vi "Clear Buffers.vi"(8 "error in (no error)":errorcluster, 11 "TDCManager":T1) -> (0 "error out":errorcluster, 3 "TDCManager":T1)   [LabVIEW 2016, in "HPTDC Driver Library.lvlib"]
uses:
  HPTDC Driver Library.lvlib
  Typedefs/TDCManager.ctl
  C:/Users/CRT Controller/CRTC Labview Application/Source/HPTDC Driver Library Folder/Library files/hptdc_net4_3.7.0_x64.dll
  hptdc_net4_3.7.0_x64.dll
panel:
  out "Succes?":bool
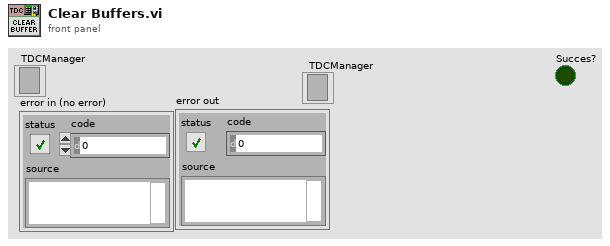
[diagram p1: front panel]
types:
  T1 = typedef "HPTDC Driver Library.lvlib/TDCManager.ctl" = refnum<k24>
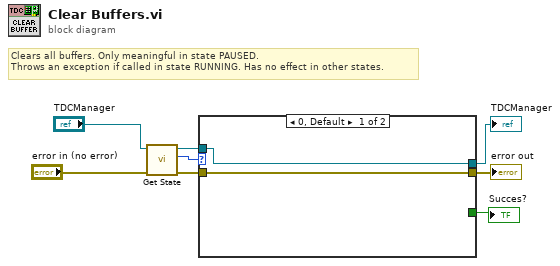
[diagram p0: block diagram]
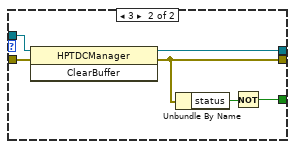
[diagram p2: hidden frame]
diagram:
  # "Clears all buffers. Only meaningful in state PAUSED.\nThrows an exception if called in state RUNNING. Has no effect in other states."
  n1 = call "Get State.vi"("error in"="error in (no error)", "TDCManager"="TDCManager") -> ("error out"=w6:errorcluster, "State"=w2:i32, "TDCManager"=w3:T1)  [unwired: 6 in, 1 out]
  n2 = case shown="0, Default" w2 {
    tunnel: w3 -> [w9 w16]
    tunnel: w6 -> [w10 w15]
    tunnel: [w10 w13] -> w8
    tunnel: [w9 w14] -> w7
    tunnel: [_ w11] -> w1
    frame 0, Default {
    }
    frame 3 {
      n3 = invoke class="HPTDCManager" method="ClearBuffer"(reference=w16, error in=w15) -> (reference out=w14:T1, error out=w13:errorcluster)  [unwired: 1 in, 1 out]
      n4 = Unbundle By Name(w13) -> ("status"=w12:bool)
      n5 = Not(x=w12) -> (.not. x?=w11:bool)
    }
  }
  "error out" <- w8
  "TDCManager" <- w7
  "Succes?" <- w1
